vi "Resolve with Error.vi"(8 "error in (no error)":errorcluster, 10 "Result":errorcluster, 11 "Promise in":refnum<class "Promise.lvclass">) -> (0 "error out":errorcluster, 1 "Future Already Completed":bool)   [LabVIEW 2017, in "Futures.lvlib" / "Promise.lvclass"]
doc: "Resolves the promise with an error.\n\nThe promise should be treated as invalid after this point and may throw errors if attempt to use it again."
uses:
  Promise.lvclass
  Promise.lvclass/Promise.ctl
  <vilib>/Utility/error.llb/Error Cluster From Error Code.vi
  Result/Result.lvclass
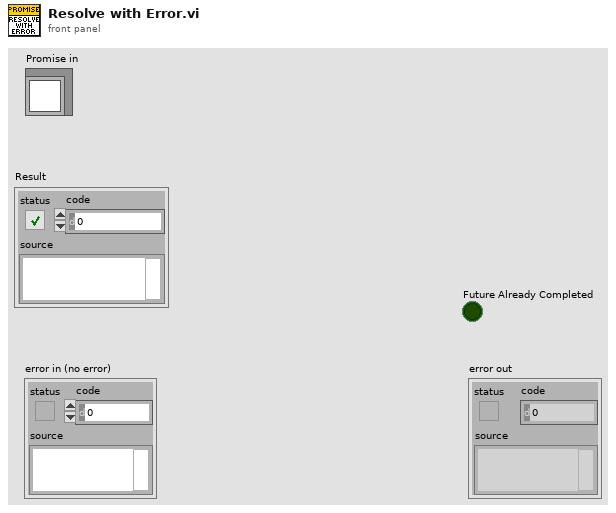
[diagram p1: front panel]
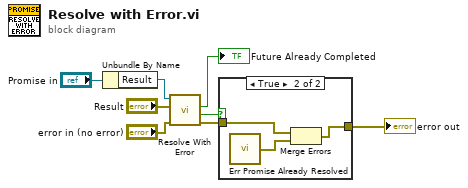
[diagram p0: block diagram]
diagram:
  n1 = Unbundle By Name("Promise in") -> ("Result"=w5:refnum<class "Result.lvclass">)
  n2 = call "Resolve With Error.vi"("error in (no error)"="error in (no error)", "Error"="Result", "Result in"=w5) -> ("error out"=w2:errorcluster, "Promise Already Resolved"=w3:bool, "Future Already Completed"=→"Future Already Completed":bool)  [unwired: 6 in]
  n3 = case shown="True" w3 {
    tunnel: w2 -> [w9 w12]
    tunnel: [w9 w10] -> w1
    frame False {
    }
    frame True {
      n4 = call "Err Promise Already Resolved.vi"() -> ("Error"=w11:errorcluster)
      n5 = Merge Errors(w12, w11) -> (w10:errorcluster)
    }
  }
  "error out" <- w1
